vi "LEP_RV_BuildSpec_PresetCheck.vi"(9 "Constant deallocation":u16(ring) items=["Out of scope", "VI end", "Application end"], 10 "Constant allocation":u16(ring) items=["First use", "VI initialization", "Application initialization", "Containing Loop"], 11 "Code generation options":T1) -> (3 "Run-Time Options":u16(ring) items=["No optimizations", "Optimize for speed", "Optimize for size", "Custom..."])   [LabVIEW 2011]
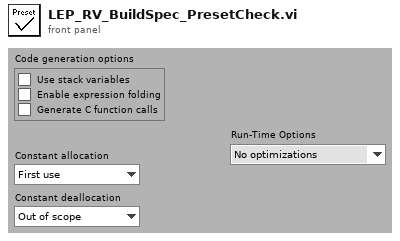
[diagram p1: front panel]
types:
  T1 = cluster{"Use stack variables":bool, "Enable expression folding":bool, "Generate C function calls":bool}
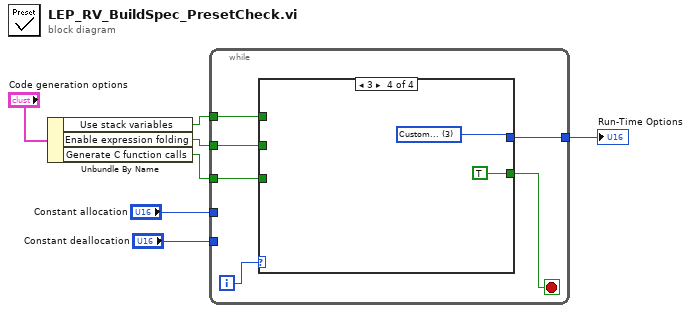
[diagram p0: block diagram]
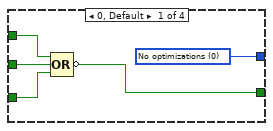
[diagram p2: hidden frame]
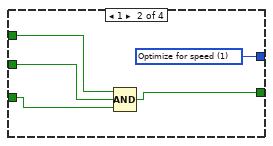
[diagram p3: hidden frame]
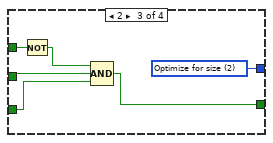
[diagram p4: hidden frame]
diagram:
  n1 = Unbundle By Name("Code generation options") -> ("Use stack variables"=w1:bool, "Enable expression folding"=w2:bool, "Generate C function calls"=w3:bool)
  n2 = while {
    tunnel: w1 -> [w12]
    tunnel: w2 -> [w11]
    tunnel: w3 -> [w10]
    tunnel: "Constant allocation" -> [_]
    tunnel: "Constant deallocation" -> [_]
    tunnel: [w8] -> w5
    i -> [w13]
    stop <- w9 stop-if-true
    n3 = case shown="3" w13 {
      tunnel: w12 -> [w18 w19 w28 _]
      tunnel: w11 -> [w17 w21 w26 _]
      tunnel: w10 -> [w16 w22 w25 _]
      tunnel: [w14 w20 w24 TRUE] -> w9
      tunnel: [w15 w23 w29 w31] -> w8
      frame 0, Default {
        w15 = u16 0 items=["No optimizations", "Optimize for speed", "Optimize for size", "Full Optimization", "Custom..."] ("Run-Time Options")
        n4 = Compound Arithmetic op=OR(w18, w17, w16) -> (invert w14:bool)
      }
      frame 1 {
        w23 = u16 1 items=["No optimizations", "Optimize for speed", "Optimize for size", "Full Optimization", "Custom..."] ("Run-Time Options")
        n5 = Compound Arithmetic op=AND(w19, w21, w22) -> (w20:bool)
      }
      frame 2 {
        w29 = u16 2 items=["No optimizations", "Optimize for speed", "Optimize for size", "Full Optimization", "Custom..."] ("Run-Time Options")
        n6 = Not(x=w28) -> (.not. x?=w27:bool)
        n7 = Compound Arithmetic op=AND(w27, w26, w25) -> (w24:bool)
      }
      frame 3 {
        w31 = u16 3 items=["No optimizations", "Optimize for speed", "Optimize for size", "Custom..."] ("Run-Time Options")
      }
    }
  }
  "Run-Time Options" <- w5
